vi "Temp_reading2_GCFS.vi"() -> ()   [LabVIEW 2024]
uses:
  <vilib>/DAQmx/create/channels.llb/DAQmx Create Channel (AI-Temperature-RTD).vi
  <vilib>/DAQmx/miscellaneous.llb/DAQmx Fill In Error Info.vi
  <vilib>/DAQmx/read.llb/DAQmx Read (Analog DBL 1Chan 1Samp).vi
panel:
  out "error out 2":errorcluster
  out "data":dbl format="%0.2f"
  out "String":string
  out "task out":refnum<k21>
  out "error out":errorcluster
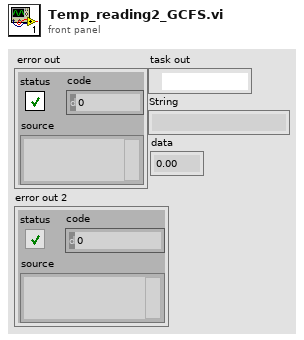
[diagram p1: front panel]
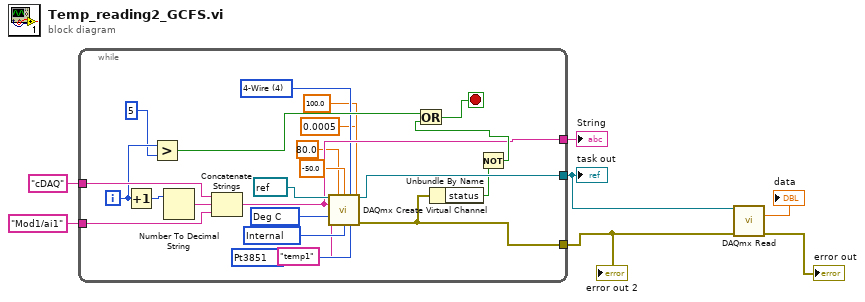
[diagram p0: block diagram]
diagram:
  n1 = while {
    tunnel: "cDAQ" -> [w30]
    tunnel: "Mod1/ai1" -> [w28]
    tunnel: [w20] -> w4
    tunnel: [w19] -> w3
    tunnel: [w16] -> w5
    i -> [w24]
    stop <- w22 stop-if-true
    w11 = 10143 items=["Deg C"=10143, "Deg F"=10144, "Kelvins"=10325, "Deg R"=10145, "From Custom Scale"=10065] ("units")
    w12 = 4 items=["2-Wire"=2, "3-Wire"=3, "4-Wire"=4] ("resistance configuration")
    w15 = 10200 items=["Internal"=10200, "External"=10167, "None"=10230] ("current excitation source")
    w25 = 10071 items=["Pt3750"=12481, "Pt3851"=10071, "Pt3911"=12482, "Pt3916"=10069, "Pt3920"=10053, "Pt3928"=12483, "Custom"=10137] ("rtd type")
    n2 = Increment(x=w24) -> (x+1=w29:i32)
    n3 = Greater?(x=w24, y=5) -> (0:w21:bool)
    n4 = Number To Decimal String(number=w29) -> (decimal integer string=w27:string)  [unwired: 1 in]
    n5 = Concatenate Strings(w30, w27, w28) -> (w16:string)
    n6 = call-poly <vilib>:"DAQmx Create Virtual Channel.vi"("task in"=refnum<k21> refnum, "maximum value"=80.0, "minimum value"=-50.0, "resistance configuration"=w12, "physical channels"=w16, "r0"=100.0, "name to assign"="temp1", "units"=w11, "current excitation value"=0.0005, "current excitation source"=w15, "rtd type"=w25) -> ("task out"=w20:refnum<k21>, "error out"=w19:errorcluster)  [unwired: 3 in]
    n7 = Unbundle By Name(w19) -> ("status"=w18:bool)
    n8 = Not(x=w18) -> (.not. x?=w17:bool)
    n9 = Or(x=w21, y=w17) -> (x .or. y?=w22:bool)
  }
  "task out" <- w4
  "String" <- w5
  "error out 2" <- w3
  n10 = call-poly <vilib>:"DAQmx Read.vi"("task/channels in"=w4, "error in"=w3) -> ("data"=→"data":dbl, "error out"=→"error out":errorcluster)  [unwired: 11 in, 1 out]
